vi "Data Message Encoding.vi"(8 "error in":errorcluster, 11 "SECS-II Class in":refnum<class "SECS-II Class.lvclass">) -> (0 "error out":errorcluster, 2 "Message Text":u8[](array[numeric]), 3 "SECS-II Class out":refnum<class "SECS-II Class.lvclass">)   [LabVIEW 2020, in "SECS Communication.lvlib" / "SECS-II Class.lvclass"]
uses:
  SECS-II Class.lvclass
  SECS-II Class.lvclass/SECS-II Class.ctl
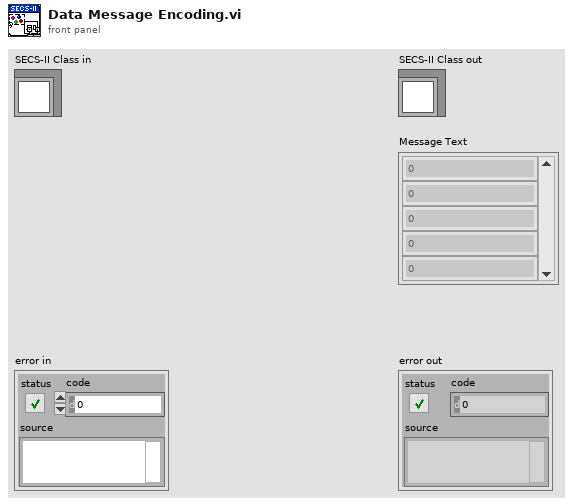
[diagram p1: front panel]
types:
  T1 = typedef "SECS Communication.lvlib/SECS-II Class.lvclass/Message Data.ctl" = cluster{"Index":i32, "Data Item Format":T2, "Format Code":T3, "Parent Index":i32, "Child Index":i32[], "Data":variant}
  T2 = typedef "SECS Communication.lvlib/SECS-II Class.lvclass/Data Item Format.ctl" = enum16{"Data Type", "Value"}
  T3 = typedef "SECS Communication.lvlib/SECS-II Class.lvclass/Format Code.ctl" = enum16{"L", "A", "B", "Boolean", "J", "I1", "I2", "I4", "I8", "U1", "U2", "U4", "U8", "F4", "F8", "Char"}
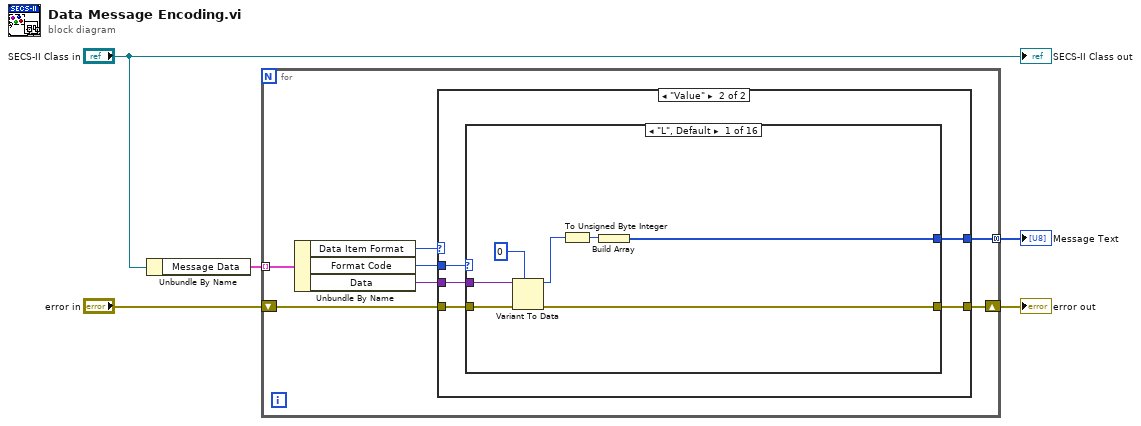
[diagram p0: block diagram]
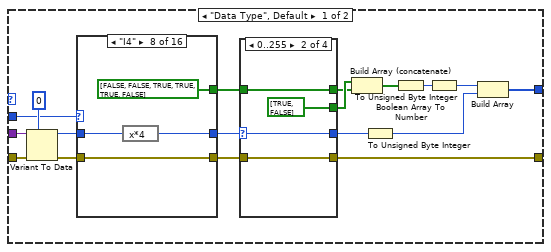
[diagram p2: hidden frame]
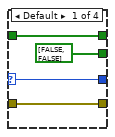
[diagram p3: hidden frame]
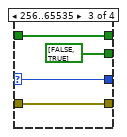
[diagram p4: hidden frame]
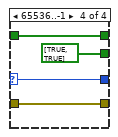
[diagram p5: hidden frame]
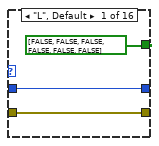
[diagram p6: hidden frame]
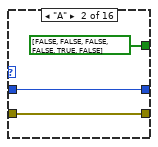
[diagram p7: hidden frame]
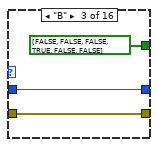
[diagram p8: hidden frame]
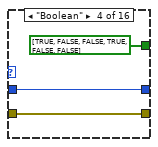
[diagram p9: hidden frame]
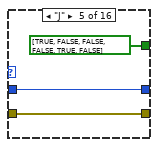
[diagram p10: hidden frame]
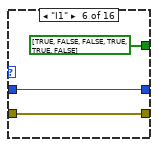
[diagram p11: hidden frame]
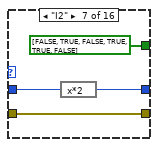
[diagram p12: hidden frame]
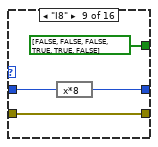
[diagram p13: hidden frame]
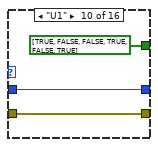
[diagram p14: hidden frame]
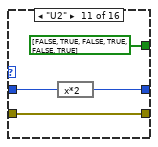
[diagram p15: hidden frame]
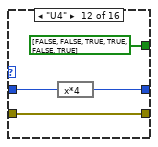
[diagram p16: hidden frame]
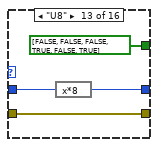
[diagram p17: hidden frame]
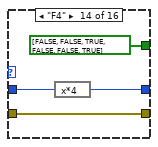
[diagram p18: hidden frame]
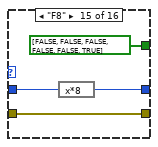
[diagram p19: hidden frame]
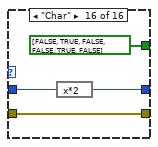
[diagram p20: hidden frame]
diagram:
  n1 = Unbundle By Name("SECS-II Class in") -> ("Message Data"=w3:T1[])
  n2 = for {
    tunnel: w3 -> [w10] mode=indexing
    tunnel: [w9] -> w4 mode=concatenating
    shift-right: [w6] -> w1
    shift-left: "error in" -> [w11]
    n3 = Unbundle By Name(w10) -> ("Data Item Format"=w12:T2, "Format Code"=w7:T3, "Data"=w8:variant)
    n4 = case shown="\"Value\"" w12 {
      tunnel: w11 -> [w29 w108]
      tunnel: [w18 w106] -> w9
      tunnel: [w17 w107] -> w6
      tunnel: w8 -> [w13 w104]
      tunnel: w7 -> [w14 w105]
      frame "Data Type", Default {
        n5 = Variant To Data(error in=w29, type=u32 0 ("Data Length"), Variant=w13) -> (data=w27:u32, error out=w28:errorcluster)
        n6 = case shown="\"I4\"" w14 {
          tunnel: w28 -> [w47 w51 w54 w57 w60 w63 w68 w72 w76 w78 w83 w87 w91 w95 w99 w103]
          tunnel: w27 -> [w48 w52 w55 w58 w61 w64 w66 w70 w74 w79 w81 w85 w89 w93 w97 w101]
          tunnel: [bool[] [FALSE, FALSE, FALSE, FALSE, FALSE, FALSE] bool[] [FALSE, FALSE, FALSE, FALSE, TRUE, FALSE] bool[] [FALSE, FALSE, FALSE, TRUE, FALSE, FALSE] bool[] [TRUE, FALSE, FALSE, TRUE, FALSE, FALSE] bool[] [TRUE, FALSE, FALSE, FALSE, TRUE, FALSE] bool[] [TRUE, FALSE, FALSE, TRUE, TRUE, FALSE] bool[] [FALSE, TRUE, FALSE, TRUE, TRUE, FALSE] bool[] [FALSE, FALSE, TRUE, TRUE, TRUE, FALSE] bool[] [FALSE, FALSE, FALSE, TRUE, TRUE, FALSE] bool[] [TRUE, FALSE, FALSE, TRUE, FALSE, TRUE] bool[] [FALSE, TRUE, FALSE, TRUE, FALSE, TRUE] bool[] [FALSE, FALSE, TRUE, TRUE, FALSE, TRUE] bool[] [FALSE, FALSE, FALSE, TRUE, FALSE, TRUE] bool[] [FALSE, FALSE, TRUE, FALSE, FALSE, TRUE] bool[] [FALSE, FALSE, FALSE, FALSE, FALSE, TRUE] bool[] [FALSE, TRUE, FALSE, FALSE, TRUE, FALSE]] -> w24
          tunnel: [w48 w52 w55 w58 w61 w64 w65 w69 w73 w79 w80 w84 w88 w92 w96 w100] -> w25
          tunnel: [w47 w51 w54 w57 w60 w63 w68 w72 w76 w78 w83 w87 w91 w95 w99 w103] -> w26
          frame "L", Default {
          }
          frame "A" {
          }
          frame "B" {
          }
          frame "Boolean" {
          }
          frame "J" {
          }
          frame "I1" {
          }
          frame "I2" {
            n7 = expression code="x*2"(w66) -> (w65:u32)
          }
          frame "I4" {
            n8 = expression code="x*4"(w70) -> (w69:u32)
          }
          frame "I8" {
            n9 = expression code="x*8"(w74) -> (w73:u32)
          }
          frame "U1" {
          }
          frame "U2" {
            n10 = expression code="x*2"(w81) -> (w80:u32)
          }
          frame "U4" {
            n11 = expression code="x*4"(w85) -> (w84:u32)
          }
          frame "U8" {
            n12 = expression code="x*8"(w89) -> (w88:u32)
          }
          frame "F4" {
            n13 = expression code="x*4"(w93) -> (w92:u32)
          }
          frame "F8" {
            n14 = expression code="x*8"(w97) -> (w96:u32)
          }
          frame "Char" {
            n15 = expression code="x*2"(w101) -> (w100:u32)
          }
        }
        n16 = case shown="0..255" w25 {
          selector: w25 -> [w31 w35 w39 w43]
          tunnel: w26 -> [w34 w38 w42 w46]
          tunnel: [w34 w38 w42 w46] -> w17
          tunnel: [bool[] [FALSE, FALSE] bool[] [TRUE, FALSE] bool[] [FALSE, TRUE] bool[] [TRUE, TRUE]] -> w23
          tunnel: w24 -> [w32 w36 w40 w44]
          tunnel: [w32 w36 w40 w44] -> w22
          tunnel: [w31 w35 w39 w43] -> w16
          frame Default {
          }
          frame 0..255 {
          }
          frame 256..65535 {
          }
          frame 65536..-1 {
          }
        }
        n17 = Build Array (concatenate)(w23, w22) -> (w21:bool[])
        n18 = To Unsigned Byte Integer(number=w16) -> (unsigned 8bit integer=w15:u8)
        n19 = Boolean Array To Number(Boolean array=w21) -> (number=w20:u32)
        n20 = To Unsigned Byte Integer(number=w20) -> (unsigned 8bit integer=w19:u8)
        n21 = Build Array(w19, w15) -> (w18:u8[])
      }
      frame "Value" {
        n22 = case shown="\"L\", Default" w105 {
          tunnel: w108 -> [w115 w121 w127 w138 w143 w149 w156 w166 w176 w184 w191 w201 w211 w221 w231 w240]
          tunnel: w104 -> [w114 w120 w126 w137 w142 w148 w155 w165 w175 w183 w190 w200 w210 w220 w230 w239]
          tunnel: [w112 w118 w125 w136 w141 w147 w154 w164 w174 w182 w189 w199 w209 w219 w229 w238] -> w107
          tunnel: [w109 w116 w122 w132 w139 w144 w150 w160 w170 w180 w185 w195 w205 w215 w225 w235] -> w106
          frame "L", Default {
            n23 = Variant To Data(error in=w115, type=0, Variant=w114) -> (data=w111:i32, error out=w112:errorcluster)
            n24 = To Unsigned Byte Integer(number=w111) -> (unsigned 8bit integer=w110:u8)
            n25 = Build Array(w110) -> (w109:u8[])
          }
          frame "A" {
            n26 = Variant To Data(error in=w121, type="", Variant=w120) -> (data=w117:string, error out=w118:errorcluster)
            n27 = String To Byte Array(string=w117) -> (unsigned byte array=w116:u8[])
          }
          frame "B" {
            n28 = Variant To Data(error in=w127, type=cluster{bool[]}[] [], Variant=w126) -> (data=w123:cluster{bool[]}[], error out=w125:errorcluster)
            n29 = for {
              tunnel: w123 -> [w131] mode=indexing
              tunnel: [w128] -> w122 mode=indexing
              n30 = Unbundle(w131) -> (w130:bool[])
              n31 = Boolean Array To Number(Boolean array=w130) -> (number=w129:u32)
              n32 = To Unsigned Byte Integer(number=w129) -> (unsigned 8bit integer=w128:u8)
            }
          }
          frame "Boolean" {
            n33 = Variant To Data(error in=w138, type=bool[] [], Variant=w137) -> (data=w134:bool[], error out=w136:errorcluster)
            n34 = Boolean To (0,1)(Boolean=w134) -> (0, 1=w133:i16[])
            n35 = To Unsigned Byte Integer(number=w133) -> (unsigned 8bit integer=w132:u8[])
          }
          frame "J" {
            n36 = Variant To Data(error in=w143, type=u8[] [], Variant=w142) -> (data=w139:u8[], error out=w141:errorcluster)
          }
          frame "I1" {
            n37 = Variant To Data(error in=w149, type=i8[] [], Variant=w148) -> (data=w145:i8[], error out=w147:errorcluster)
            n38 = To Unsigned Byte Integer(number=w145) -> (unsigned 8bit integer=w144:u8[])
          }
          frame "I2" {
            n39 = Variant To Data(error in=w156, type=i16[] [], Variant=w155) -> (data=w152:i16[], error out=w154:errorcluster)
            n40 = for {
              tunnel: w152 -> [w159] mode=indexing
              tunnel: u8[] [] -> [w158]
              tunnel: [w157] -> w150 mode=concatenating
              n41 = Type Cast(type=w158, x=w159) -> (*(type *) &x=w157:u8[])
            }
          }
          frame "I4" {
            n42 = Variant To Data(error in=w166, type=i32[] [], Variant=w165) -> (data=w162:i32[], error out=w164:errorcluster)
            n43 = for {
              tunnel: w162 -> [w169] mode=indexing
              tunnel: u8[] [] -> [w168]
              tunnel: [w167] -> w160 mode=concatenating
              n44 = Type Cast(type=w168, x=w169) -> (*(type *) &x=w167:u8[])
            }
          }
          frame "I8" {
            n45 = Variant To Data(error in=w176, type=i64[] [], Variant=w175) -> (data=w172:i64[], error out=w174:errorcluster)
            n46 = for {
              tunnel: w172 -> [w179] mode=indexing
              tunnel: u8[] [] -> [w178]
              tunnel: [w177] -> w170 mode=concatenating
              n47 = Type Cast(type=w178, x=w179) -> (*(type *) &x=w177:u8[])
            }
          }
          frame "U1" {
            n48 = Variant To Data(error in=w184, type=u8[] [], Variant=w183) -> (data=w180:u8[], error out=w182:errorcluster)
          }
          frame "U2" {
            n49 = Variant To Data(error in=w191, type=u16[] [], Variant=w190) -> (data=w187:u16[], error out=w189:errorcluster)
            n50 = for {
              tunnel: w187 -> [w194] mode=indexing
              tunnel: u8[] [] -> [w193]
              tunnel: [w192] -> w185 mode=concatenating
              n51 = Type Cast(type=w193, x=w194) -> (*(type *) &x=w192:u8[])
            }
          }
          frame "U4" {
            n52 = Variant To Data(error in=w201, type=u32[] [], Variant=w200) -> (data=w197:u32[], error out=w199:errorcluster)
            n53 = for {
              tunnel: w197 -> [w204] mode=indexing
              tunnel: u8[] [] -> [w203]
              tunnel: [w202] -> w195 mode=concatenating
              n54 = Type Cast(type=w203, x=w204) -> (*(type *) &x=w202:u8[])
            }
          }
          frame "U8" {
            n55 = Variant To Data(error in=w211, type=u64[] [], Variant=w210) -> (data=w207:u64[], error out=w209:errorcluster)
            n56 = for {
              tunnel: w207 -> [w214] mode=indexing
              tunnel: u8[] [] -> [w213]
              tunnel: [w212] -> w205 mode=concatenating
              n57 = Type Cast(type=w213, x=w214) -> (*(type *) &x=w212:u8[])
            }
          }
          frame "F4" {
            n58 = Variant To Data(error in=w221, type=sgl[] [], Variant=w220) -> (data=w217:sgl[], error out=w219:errorcluster)
            n59 = for {
              tunnel: w217 -> [w224] mode=indexing
              tunnel: u8[] [] -> [w223]
              tunnel: [w222] -> w215 mode=concatenating
              n60 = Type Cast(type=w223, x=w224) -> (*(type *) &x=w222:u8[])
            }
          }
          frame "F8" {
            n61 = Variant To Data(error in=w231, type=dbl[] [], Variant=w230) -> (data=w227:dbl[], error out=w229:errorcluster)
            n62 = for {
              tunnel: w227 -> [w234] mode=indexing
              tunnel: u8[] [] -> [w233]
              tunnel: [w232] -> w225 mode=concatenating
              n63 = Type Cast(type=w233, x=w234) -> (*(type *) &x=w232:u8[])
            }
          }
          frame "Char" {
            n64 = Variant To Data(error in=w240, type="", Variant=w239) -> (data=w236:string, error out=w238:errorcluster)
            n65 = String To Byte Array(string=w236) -> (unsigned byte array=w235:u8[])
          }
        }
      }
    }
  }
  "error out" <- w1
  "Message Text" <- w4
  "SECS-II Class out" <- "SECS-II Class in"
